vi "Build Coffee Shop.vi"(8 "error in (no error)":errorcluster) -> (0 "error out":errorcluster, 3 "Coffee Shop Out":refnum<class "Coffee Shop.lvclass">)   [LabVIEW 2020, in "Coffee Shop.lvclass"]
uses:
  Coffee Shop.lvclass
  Work Dispatcher/Work Dispatcher.lvclass
  C:/Users/anton/Documents/GitHub/Triarc-Examples/Coffee Shop/Process Job/Job Handler.lvclass
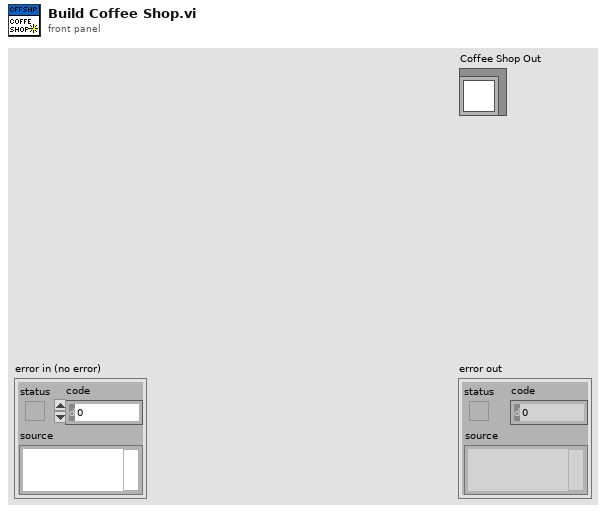
[diagram p1: front panel]
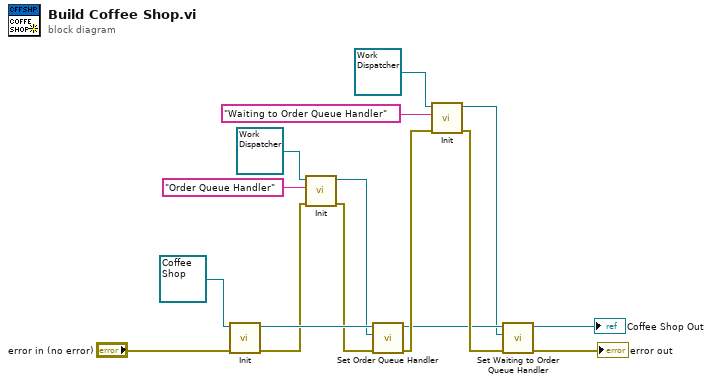
[diagram p0: block diagram]
diagram:
  n1 = call-dynamic "Init.vi"("error in (no error)"="error in (no error)", "Process In"=refnum<class "Coffee Shop.lvclass"> refnum ("Coffee Shop.lvclass")) -> ("error out"=w10:errorcluster, "Process Out"=w14:refnum<class "Coffee Shop.lvclass">)  [unwired: 8 in]
  n2 = call-dynamic "Init.vi"("error in (no error)"=w10, "Name"="Order Queue Handler", "Process In"=refnum<class "Work Dispatcher.lvclass"> refnum ("Work Dispatcher.lvclass")) -> ("error out"=w9:errorcluster, "Process Out"=w3:refnum<class "Work Dispatcher.lvclass">)  [unwired: 7 in]
  n3 = call "Set Order Queue Handler.vi"("error in (no error)"=w9, "Order Queue Handler"=w3, "Coffee Shop In"=w14) -> ("error out"=w7:errorcluster, "Coffee Shop Out"=w5:refnum<class "Coffee Shop.lvclass">)  [unwired: 7 in]
  n4 = call-dynamic "Init.vi"("error in (no error)"=w7, "Name"="Waiting to Order Queue Handler", "Process In"=refnum<class "Work Dispatcher.lvclass"> refnum ("Work Dispatcher.lvclass")) -> ("error out"=w6:errorcluster, "Process Out"=w4:refnum<class "Work Dispatcher.lvclass">)  [unwired: 7 in]
  n5 = call "Set Waiting to Order Queue Handler.vi"("error in (no error)"=w6, "Waiting To Order Queue Handler"=w4, "Coffee Shop In"=w5) -> ("error out"=→"error out":errorcluster, "Coffee Shop Out"=→"Coffee Shop Out":refnum<class "Coffee Shop.lvclass">)  [unwired: 7 in]
